vi "SpecPage.vi"(10 "Spec Page Interface":T1, 11 "MetaDataObj in":refnum<class "MetaDataObj.lvclass">) -> (3 "MetaDataObj out":refnum<class "MetaDataObj.lvclass">)   [LabVIEW 2021, in "CIF_NewPluginTemplate.lvclass"]
uses:
  CIF_NewPluginTemplate.lvclass
  <resource>/dialog/NewProjectWizard/Spec Page Interface.ctl
  <resource>/dialog/NewProjectWizard/MetaDataObj/MetaDataObj.lvclass
  <resource>/dialog/NewProjectWizard/MetaDataObj/MetaDataObj.lvclass/MetaDataObj.ctl
  <resource>/dialog/NewProjectWizard/MetaDataObj/Accessors/Read Overlay Pixmap.vi
  <resource>/dialog/NewProjectWizard/MetaDataObj/Accessors/Write Overlay Pixmap.vi
  <resource>/dialog/NewProjectWizard/MetaDataObj/Accessors/Write File Prefix.vi
  <resource>/dialog/NewProjectWizard/MetaDataObj/Accessors/Write Project Name.vi
  <resource>/dialog/NewProjectWizard/MetaDataObj/Accessors/Write Project Root.vi
  <resource>/dialog/NewProjectWizard/MetaDataObj/Accessors/Read Hide Prefix.vi
  <resource>/dialog/NewProjectWizard/MetaDataObj/Accessors/Read Hide Icon Overlay.vi
  <vilib>/LabVIEW Icon API/lv_icon/Classes/Icon/Icon.lvclass
  CIF_NewPluginTemplate.lvclass/CIF_NewPluginTemplate.ctl
  <resource>/dialog/NewProjectWizard/Icon Overlay/NI_NPW_Icon Overlay.lvlib
  <vilib>/LabVIEW Icon API/LabVIEW Icon API.lvlib
  C:/Program Files/National Instruments/LabVIEW 2021/resource/dialog/NewProjectWizard/MetaDataObj/MetaDataObj.lvclass
  D:/dev/CIF-LVCore/src/CIFUtilities/Scripting/Plugin Generator/CIF_NewPluginTemplate/CIF_NewPluginTemplate.lvclass
panel:
  in  "Project Name":string
  in  "Project Root":path
  in  "File Name Prefix (Optional)":string
  out "Modified Icon":picture
  in  "Sample Icon":picture
  out "Overlay (picture)":picture
  in  "Edit Icon Overlay":bool
  # "Modify VI Icons"
  # "+"
  # "="
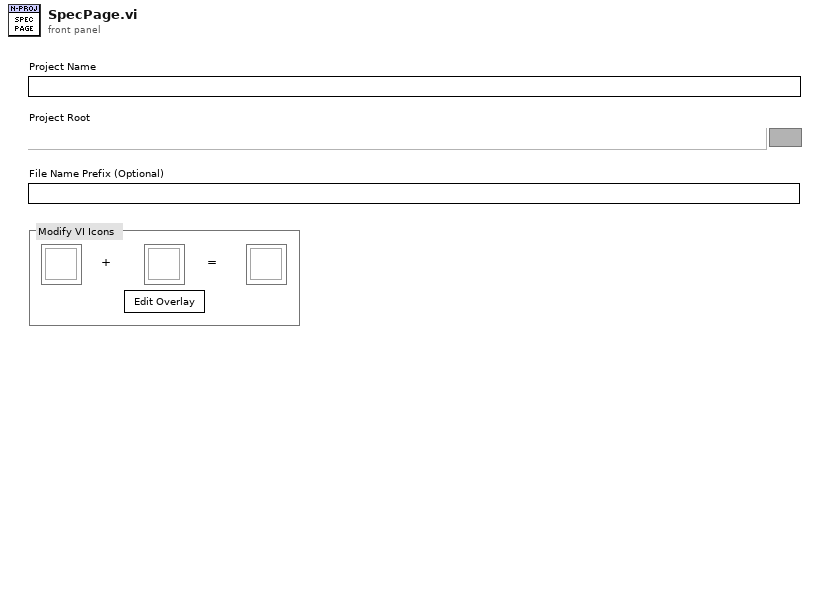
[diagram p1: front panel]
types:
  T1 = typedef "Spec Page Interface.ctl" = cluster{"\"Tab Forward To\" Refnum":refnum<vi>, "\"Tab Backward To\" Refnum":refnum<vi>, "Errors":refnum<user-event>, "Quit":refnum<user-event>}
  T2 = typedef "imagedata.ctl" = cluster{"image type":i32, "image depth":i32, "image":u8[], "mask":u8[], "colors":u32[], "Rectangle":cluster{"left":i16, "top":i16, "right":i16, "bottom":i16}}
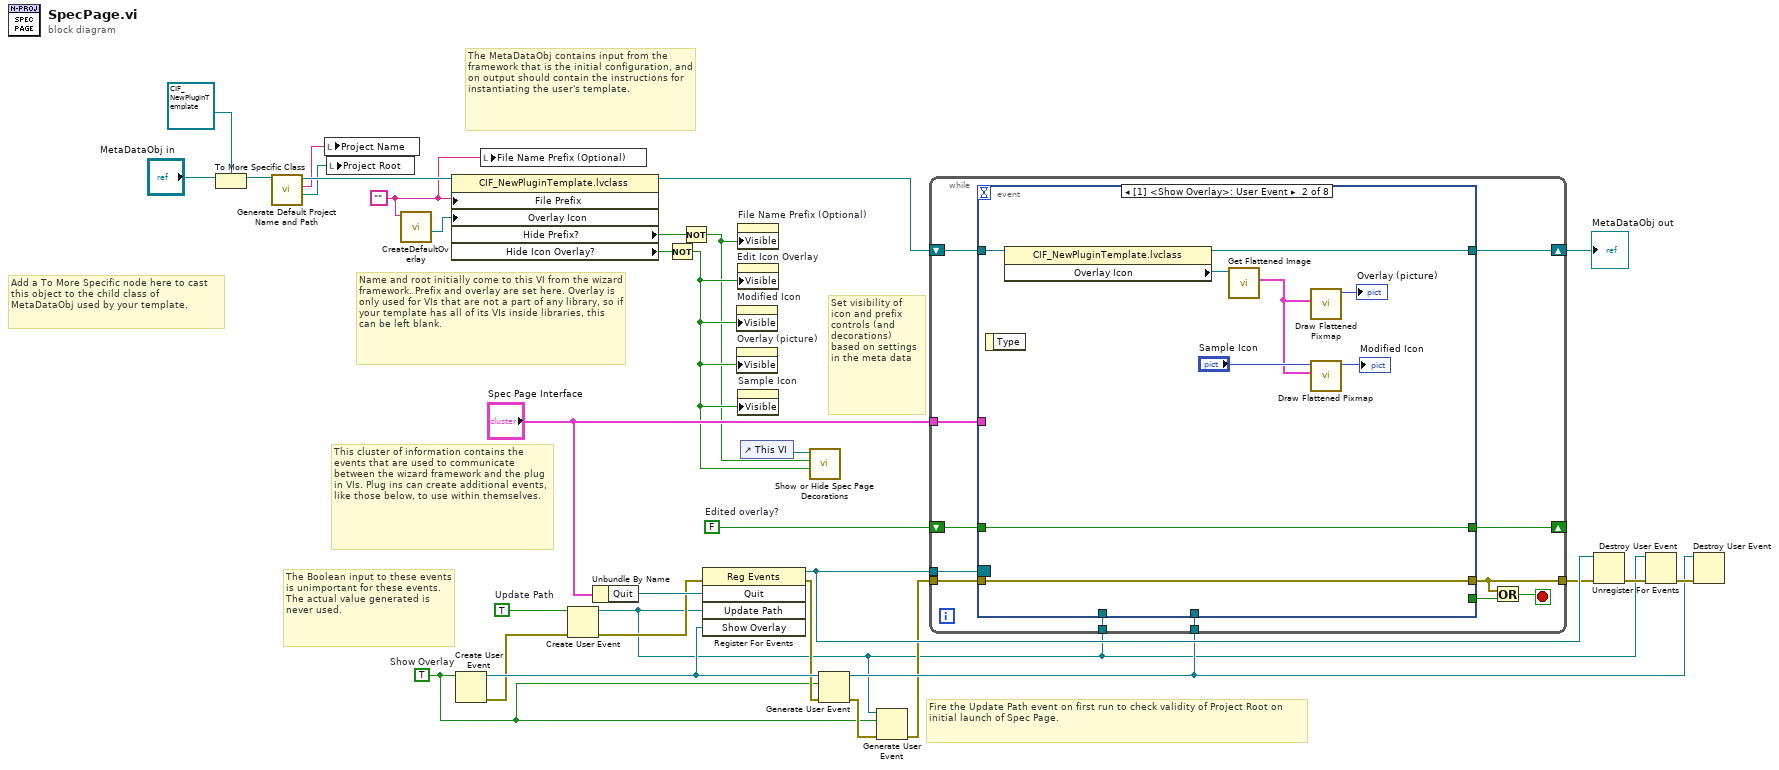
[diagram p0: block diagram]
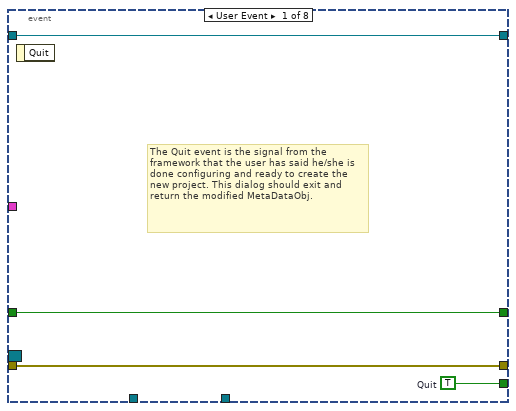
[diagram p2: hidden frame]
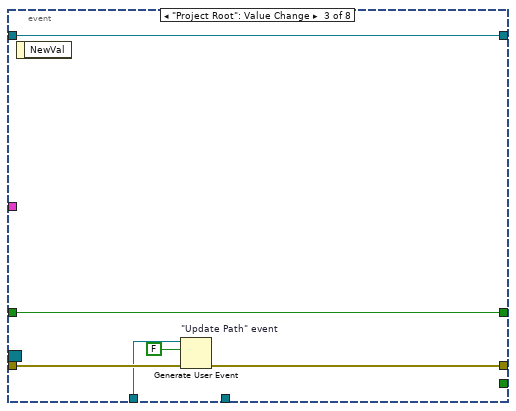
[diagram p3: hidden frame]
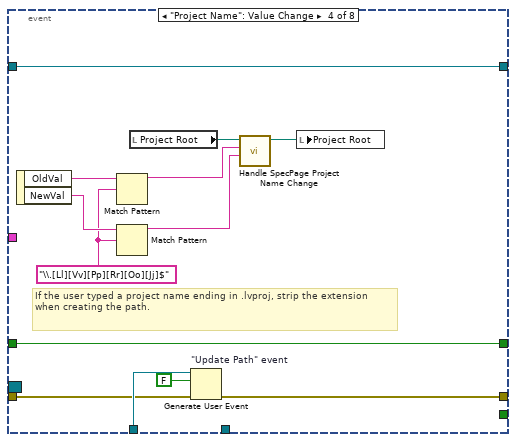
[diagram p4: hidden frame]
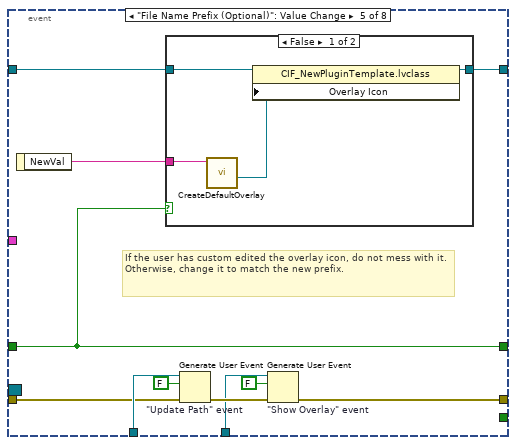
[diagram p5: hidden frame]
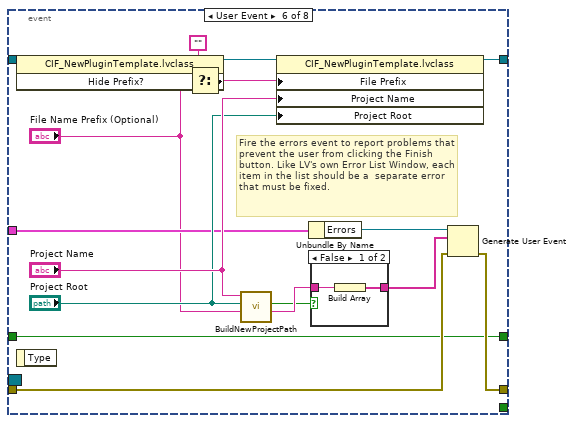
[diagram p7: hidden frame]
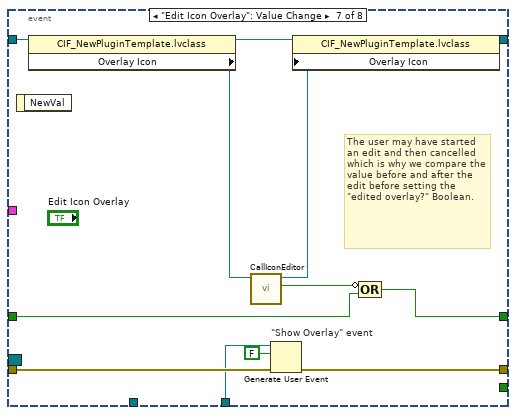
[diagram p9: hidden frame]
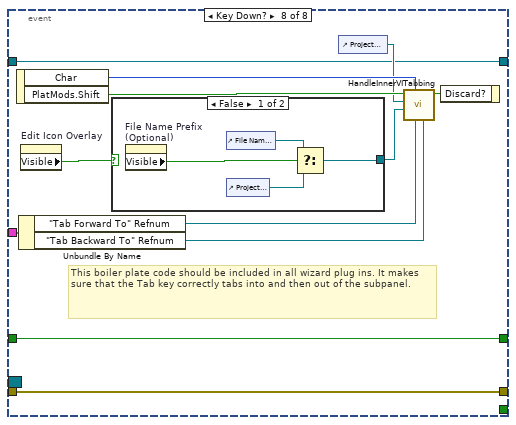
[diagram p10: hidden frame]
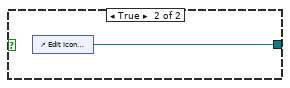
[diagram p11: hidden frame]
diagram:
  w5 = ""
  w23 = FALSE  # Edited overlay?
  w16 = TRUE  # Show Overlay
  w28 = TRUE  # Update Path
  # "Set visibility of icon and prefix controls (and decorations) based on settings in the meta data"
  # "Fire the Update Path event on first run to check validity of Project Root on initial launch of Spec Page."
  # "The Boolean input to these events is unimportant for these events. The actual value generated is never used."
  # "This cluster of information contains the events that are used to communicate between the wizard framework and the plug in VIs. Plug ins can create additional events, like those below, to use within themselves."
  # "The MetaDataObj contains input from the framework that is the initial configuration, and on output should contain the instructions for instantiating the user's template."
  # "Add a To More Specific node here to cast this object to the child class of MetaDataObj used by your template."
  # "Name and root initially come to this VI from the wizard framework. Prefix and overlay are set here. Overlay is only used for VIs that are not a part of any library, so if your template has all of its VIs inside libraries, this can be left blank."
  n1 = To More Specific Class(target class=refnum<class "CIF_NewPluginTemplate.lvclass"> refnum ("CIF_NewPluginTemplate.lvclass"), reference="MetaDataObj in") -> (specific class reference=w3:refnum<class "CIF_NewPluginTemplate.lvclass">)  [unwired: 1 in, 1 out]
  n2 = call <resource>:"Generate Default Project Name and Path.vi"("DNL_MetaDataObj in"=w3) -> ("Project Root"=w6:path, "Project Name"=w7:string, "DNL_MetaDataObj out"=w8:refnum<class "CIF_NewPluginTemplate.lvclass">)  [unwired: 8 in]
  n3 = local write "Project Name"(w7) -> ()
  n4 = local write "Project Root"(w6) -> ()
  n5 = call <resource>:"CreateDefaultOverlay.vi"("File Prefix"=w5) -> ("Overlay Icon"=w1:refnum<class "Icon.lvclass">)  [unwired: 8 in, 2 out]
  n6 = property class="CIF_NewPluginTemplate.lvclass"(reference=w8, "File Prefix"=w5, "Overlay Icon"=w1) -> (reference out=w14:refnum<class "CIF_NewPluginTemplate.lvclass">, "Hide Prefix?"=w13:bool, "Hide Icon Overlay?"=w12:bool)  [unwired: 1 in, 1 out]
  n7 = Create User Event(user event datatype=w16) -> (user event=w22:refnum<user-event>, error out=w19:errorcluster)  [unwired: 1 in]
  n8 = local write "File Name Prefix (Optional)"(w5) -> ()
  n9 = Create User Event(user event datatype=w28, error in=w19) -> (user event=w15:refnum<user-event>, error out=w27:errorcluster)
  n10 = Unbundle By Name("Spec Page Interface") -> ("Quit"=w32:refnum<user-event>)
  n11 = Not(x=w12) -> (.not. x?=w10:bool)
  n12 = Not(x=w13) -> (.not. x?=w9:bool)
  n13 = register-events(error in=w27, w32, w15, w22) -> (reference out=w31:refnum<event-registration>, error out=w20:errorcluster)  [unwired: 1 in]
  n14 = property on="Modified Icon" class="Pict"("Visible"=w10) -> ()  [unwired: 2 in, 2 out]
  n15 = property on="Overlay (picture)" class="Pict"("Visible"=w10) -> ()  [unwired: 2 in, 2 out]
  n16 = property on="File Name Prefix (Optional)" class="Str"("Visible"=w9) -> ()  [unwired: 2 in, 2 out]
  n17 = property on="Edit Icon Overlay" class="Bool"("Visible"=w10) -> ()  [unwired: 2 in, 2 out]
  n18 = property on="Sample Icon" class="Pict"("Visible"=w10) -> ()  [unwired: 2 in, 2 out]
  n19 = control-ref of="This VI"() -> (w11:refnum<vi>)
  n20 = call <resource>:"Show or Hide Spec Page Decorations.vi"("Icon Visible"=w10, "Prefix Visible"=w9, "Spec Page refnum"=w11) -> ()  [unwired: 9 in]
  n21 = Generate User Event(user event=w22, event data cluster=w16, error in=w20) -> (user event out=w21:refnum<user-event>, error out=w18:errorcluster)  [unwired: 1 in]
  n22 = Generate User Event ("\"Update Path\" event")(user event=w15, event data cluster=w16, error in=w18) -> (error out=w17:errorcluster)  [unwired: 1 in, 1 out]
  n23 = while {
    tunnel: "Spec Page Interface" -> [w42]
    shift-right: [w41] -> w25
    shift-left: w14 -> [w40]
    tunnel: w31 -> [w44]
    tunnel: w17 -> [w43]
    tunnel: [w37] -> w29
    tunnel: w15 -> [w36]
    tunnel: w21 -> [w35]
    shift-right: [w33] -> _
    shift-left: w23 -> [w34]
    stop <- w39 stop-if-true
    n24 = event shown="[1] <Show Overlay>: User Event" {
      selector: w44 -> [_ _ _ _ _ _ _ _]
      dyn-events: _ -> [_ _ _ _ _ _ _ _]
      timeout: _ -> [_ _ _ _ _ _ _ _]
      tunnel: w42 -> [_ _ _ _ _ w103 _ w131]
      tunnel: [w48 _ _ _ _ _ _ _] -> w38
      tunnel: [w47 w57 w61 w72 w79 w101 w118 w128] -> w37
      tunnel: w43 -> [w47 w57 w62 w73 w85 w102 w119 w128]
      tunnel: [w46 w52 w63 w69 w82 w99 w123 w127] -> w41
      tunnel: w40 -> [w46 w53 w63 w69 w83 w100 w122 w127]
      tunnel: w36 -> [_ _ w60 w74 w87 _ _ _]
      tunnel: w35 -> [_ _ _ _ w78 _ w117 _]
      tunnel: w34 -> [w45 w51 w58 w70 w77 w98 w116 w126]
      tunnel: [w45 w51 w58 w70 w77 w98 w115 w126] -> w33
      event User Event {
        w48 = TRUE  # Quit
        # "The Quit event is the signal from the framework that the user has said he/she is done configuring and ready to create the new project. This dialog should exit and return the modified MetaDataObj."
        n25 = event-data() -> ()  [unwired: 1 in, 1 out]
      }
      event User Event {
        n26 = event-data() -> ()  [unwired: 1 in, 1 out]
        n27 = property class="CIF_NewPluginTemplate.lvclass"(reference=w53) -> (reference out=w52:refnum<class "CIF_NewPluginTemplate.lvclass">, "Overlay Icon"=w50:refnum<class "Icon.lvclass">)  [unwired: 1 in, 1 out]
        n28 = call <vilib>:"Get Flattened Image.vi"("lv_icon.lvlib:Icon.lvclass in"=w50) -> ("Color Image"=w49:T2)  [unwired: 7 in, 3 out]
        n29 = call <vilib>:"Draw Flattened Pixmap.vi"("image data"=w49) -> ("new picture"=→"Overlay (picture)":picture)  [unwired: 8 in]
        n30 = call <vilib>:"Draw Flattened Pixmap.vi"("image data"=w49, "picture"="Sample Icon") -> ("new picture"=→"Modified Icon":picture)  [unwired: 7 in]
      }
      event "Project Root": Value Change {
        n31 = event-data() -> ()  [unwired: 1 in, 1 out]
        n32 = Generate User Event "\"Update Path\" event"(user event=w60, event data cluster=FALSE ("event data"), error in=w62) -> (error out=w61:errorcluster)  [unwired: 1 in, 1 out]
      }
      event "Project Name": Value Change {
        w64 = "\\.[Ll][Vv][Pp][Rr][Oo][Jj]$" ("regular expression")
        # "If the user typed a project name ending in .lvproj, strip the extension when creating the path."
        n33 = event-data() -> ("OldVal"=w66:string, "NewVal"=w68:string)  [unwired: 1 in]
        n34 = Match Pattern(string=w66, regular expression=w64) -> (before substring=w65:string)  [unwired: 1 in, 3 out]
        n35 = Match Pattern(string=w68, regular expression=w64) -> (before substring=w67:string)  [unwired: 1 in, 3 out]
        n36 = local read "Project Root"() -> (w76:path)
        n37 = Generate User Event "\"Update Path\" event"(user event=w74, event data cluster=FALSE ("event data"), error in=w73) -> (error out=w72:errorcluster)  [unwired: 1 in, 1 out]
        n38 = call <resource>:"Handle SpecPage Project Name Change.vi"("Project Name New Value"=w67, "Project Name Old Value"=w65, "Project Root in"=w76) -> ("Project Root out"=w75:path)  [unwired: 8 in]
        n39 = local write "Project Root"(w75) -> ()
      }
      event "File Name Prefix (Optional)": Value Change {
        # "If the user has custom edited the overlay icon, do not mess with it. Otherwise, change it to match the new prefix."
        n40 = event-data() -> ("NewVal"=w84:string)  [unwired: 1 in]
        n41 = case shown="False" w77 {
          tunnel: w84 -> [w91 _]
          tunnel: w83 -> [w90 w92]
          tunnel: [w89 w92] -> w82
          frame False {
            n42 = call <resource>:"CreateDefaultOverlay.vi"("File Prefix"=w91) -> ("Overlay Icon"=w88:refnum<class "Icon.lvclass">)  [unwired: 8 in, 2 out]
            n43 = property class="CIF_NewPluginTemplate.lvclass"(reference=w90, "Overlay Icon"=w88) -> (reference out=w89:refnum<class "CIF_NewPluginTemplate.lvclass">)  [unwired: 1 in, 1 out]
          }
          frame True {
          }
        }
        n44 = Generate User Event "\"Update Path\" event"(user event=w87, event data cluster=FALSE ("event data"), error in=w85) -> (error out=w80:errorcluster)  [unwired: 1 in, 1 out]
        n45 = Generate User Event "\"Show Overlay\" event"(user event=w78, event data cluster=FALSE ("event data"), error in=w80) -> (error out=w79:errorcluster)  [unwired: 1 in, 1 out]
      }
      event User Event {
        # "Fire the errors event to report problems that prevent the user from clicking the Finish button. Like LV's own Error List Window, each item in the list should be a  separate error that must be fixed."
        n46 = property class="CIF_NewPluginTemplate.lvclass"(reference=w100) -> (reference out=w97:refnum<class "CIF_NewPluginTemplate.lvclass">, "Hide Prefix?"=w95:bool)  [unwired: 1 in, 1 out]
        n47 = event-data() -> ()  [unwired: 1 in, 1 out]
        n48 = Select(t="", s=w95, f="File Name Prefix (Optional)") -> (s? t:f=w94:string)
        n49 = call <resource>:"BuildNewProjectPath.vi"("File Prefix"="File Name Prefix (Optional)", "Project Root"="Project Root", "Project Name"="Project Name") -> ("Error Message"=w106:string, "Valid?"=w104:bool)  [unwired: 6 in, 1 out]
        n50 = property class="CIF_NewPluginTemplate.lvclass"(reference=w97, "File Prefix"=w94, "Project Name"="Project Name", "Project Root"="Project Root") -> (reference out=w99:refnum<class "CIF_NewPluginTemplate.lvclass">)  [unwired: 1 in, 1 out]
        n51 = Unbundle By Name(w103) -> ("Errors"=w109:refnum<user-event>)
        n52 = case shown="False" w104 {
          tunnel: w106 -> [w111 _]
          tunnel: [w110 _] -> w105
          frame False {
            n53 = Build Array(w111) -> (w110:string[])
          }
          frame True {
          }
        }
        n54 = Generate User Event(user event=w109, event data cluster=w105, error in=w102) -> (error out=w101:errorcluster)  [unwired: 1 in, 1 out]
      }
      event "Edit Icon Overlay": Value Change {
        # "The user may have started an edit and then cancelled which is why we compare the value before and after the edit before setting the \"edited overlay?\" Boolean."
        n55 = event-data() -> ()  [unwired: 1 in, 1 out]
        n56 = property class="CIF_NewPluginTemplate.lvclass"(reference=w122) -> (reference out=w121:refnum<class "CIF_NewPluginTemplate.lvclass">, "Overlay Icon"=w114:refnum<class "Icon.lvclass">)  [unwired: 1 in, 1 out]
        n57 = call <resource>:"CallIconEditor.vi"("Icon in"=w114) -> ("Canceled?"=w112:bool, "Icon out"=w113:refnum<class "Icon.lvclass">)  [unwired: 9 in]
        n58 = Generate User Event "\"Show Overlay\" event"(user event=w117, event data cluster=FALSE ("event data"), error in=w119) -> (error out=w118:errorcluster)  [unwired: 1 in, 1 out]
        n59 = property class="CIF_NewPluginTemplate.lvclass"(reference=w121, "Overlay Icon"=w113) -> (reference out=w123:refnum<class "CIF_NewPluginTemplate.lvclass">)  [unwired: 1 in, 1 out]
        n60 = Compound Arithmetic op=OR(invert w112, w116) -> (w115:bool)
      }
      event Key Down? {
        # "This boiler plate code should be included in all wizard plug ins. It makes sure that the Tab key correctly tabs into and then out of the subpanel."
        n61 = event-data() -> ("Char"=w134:i16, "PlatMods.Shift"=w133:bool)  [unwired: 1 in]
        n62 = Unbundle By Name(w131) -> ("\"Tab Forward To\" Refnum"=w130:refnum<vi>, "\"Tab Backward To\" Refnum"=w129:refnum<vi>)
        n63 = property on="Edit Icon Overlay" class="Bool"() -> ("Visible"=w125:bool)  [unwired: 2 in, 2 out]
        n64 = case shown="False" w125 {
          tunnel: [w136 w140] -> w124
          frame False {
            n65 = property on="File Name Prefix (Optional)" class="Str"() -> ("Visible"=w139:bool)  [unwired: 2 in, 2 out]
            n66 = control-ref of="File Name Prefix (Optional)"() -> (w138:refnum<vi>)
            n67 = control-ref of="Project Root"() -> (w137:refnum<vi>)
            n68 = Select(t=w138, s=w139, f=w137) -> (s? t:f=w136:refnum<vi>)
          }
          frame True {
            n69 = control-ref of="Edit Icon Overlay"() -> (w140:refnum<vi>)
          }
        }
        n70 = control-ref of="Project Name"() -> (w132:refnum<vi>)
        n71 = call <resource>:"HandleInnerVITabbing.vi"("Tab Backward To"=w129, "Tab Forward To"=w130, "Char"=w134, "Last Control"=w124, "First Control"=w132, "Shift"=w133) -> ("Discard"=w135:bool)  [unwired: 5 in]
        n72 = event-data("Discard?"=w135) -> ()  [unwired: 1 in, 1 out]
      }
    }
    n73 = Or(x=w37, y=w38) -> (x .or. y?=w39:bool)
  }
  "MetaDataObj out" <- w25
  n74 = Unregister For Events(event registration refnum=w31, error in=w29) -> (error out=w26:errorcluster)
  n75 = Destroy User Event(user event=w15, error in=w26) -> (error out=w24:errorcluster)
  n76 = Destroy User Event(user event=w21, error in=w24) -> ()  [unwired: 1 out]
